vi "main.vi"() -> ()   [LabVIEW 2015]
uses:
  <vilib>/Utility/error.llb/DialogType.ctl
panel:
  out "d1_B2n":dbl
  out "d1_B1n":dbl
  out "d1_A2n":dbl
  out "d1_A1n":dbl
  out "con1":refnum<k5>
  in  "Tab Control":enum32{"ИЗМЕРЕНИЯ", "НАСТРОЙКИ"}(tab)
  out "d1_A1":string="-"
  out "d1_A2":string
  out "d1_B1":string="-"
  out "d1_B2":string
  in  "1_A1":bool=TRUE
  in  "1_A2":bool=TRUE
  in  "1_B1":bool=TRUE
  in  "1_B2":bool=TRUE
  out "con status 1":bool
  out "con2":refnum<k5>
  out "con status 2":bool
  in  "2_B1":bool=TRUE
  out "d2_B1":string="\r\n"
  in  "2_B2":bool=TRUE
  out "d2_B2":string="\r\n"
  in  "2_A2":bool=TRUE
  out "d2_A2":string
  in  "2_A1":bool=TRUE
  out "d2_A1":string
  out "d2_B2n":dbl
  out "d2_B1n":dbl
  out "d2_A2n":dbl
  out "d2_A1n":dbl
  out "refnum out":refnum<file>
  in  "P max lp":dbl=1000.0 min=0.0 max=10000000.0 step=1e-06 format="%3.2e"
  in  "P min lp":dbl min=0.0 max=10000000.0 step=1e-06 format="%3.2e"
  in  "Autoscale 2":bool=TRUE
  in  "P max hp":dbl=1000.0 min=0.0 max=10000000.0 step=1e-06 format="%3.2e"
  in  "P min hp":dbl min=0.0 max=10000000.0 step=1e-06 format="%3.2e"
  in  "Autoscale 1":bool=TRUE
  in  "port1":u16=4001
  in  "D1 IP":string="192.168.127.253"
  in  "D2 IP":string="192.168.127.253"
  in  "port2":u16=4001
  in  "d2_B2s":enum32{"Radio Selection 1", "Radio Selection 2"}(radio)
  in  "d2_B1s":enum32{"Radio Selection 1", "Radio Selection 2"}(radio)
  in  "d2_A2s":enum32{"Radio Selection 1", "Radio Selection 2"}(radio)
  in  "d2_A1s":enum32{"Radio Selection 1", "Radio Selection 2"}(radio)
  in  "d1_B2s":enum32{"Radio Selection 1", "Radio Selection 2"}(radio)
  in  "d1_B1s":enum32{"Radio Selection 1", "Radio Selection 2"}(radio)
  in  "d1_A2s":enum32{"Radio Selection 1", "Radio Selection 2"}(radio)
  in  "d1_A1s":enum32{"Radio Selection 1", "Radio Selection 2"}(radio)
  in  "stop":bool
  in  "xScale +":bool
  in  "xScale -":bool
  in  "Добавить время":dbl(ring)=300.0 items=["1 мин."=60.0, "5 мин."=300.0, "20 мин."=1200.0]
  out "мин.":string="1"
  out "часы":string="0"
  out "Graphs hP":dynamicdata(graph) caption="Высокий вакуум, мБар"
  out "сек.":string="0"
  out "Сутки":string
  out "Graphs lP":dynamicdata(graph) caption="Низкий вакуум, мБар"
  # "D1"
  # "A1"
  # "A2"
  # "B1"
  # "B2"
  # "D2"
  # "A1"
  # "A2"
  # "B1"
  # "B2"
  # "Высокий вакуум"
  # "Низкий вакуум"
  # "Отображение на графиках"
  # "Высокий"
  # "Низкий"
  # "D2 B2"
  # "D2 B1"
  # "D2 A2"
  # "D2 A1"
  # "D1 B2"
  # "D1 B1"
  # "D1 A2"
  # "D1 A1"
  # "Интервал графиков"
  # ":"
types:
  T1 = typedef "DialogType.ctl" = u16
  T2 = typedef "RWC_Actions.ctl" = enum16{"Read", "Write", "Read and Create"}
  T3 = typedef "LVDateTimeRec.ctl" = cluster{"fractional second":dbl, "second":i32, "minute":i32, "hour":i32, "day of month":i32, "month":i32, "year":i32, "day of week":i32, "day of year":i32, "DST":i32}
  T4 = enum8{"Enabled", "Disabled", "Disabled and Grayed Out"}
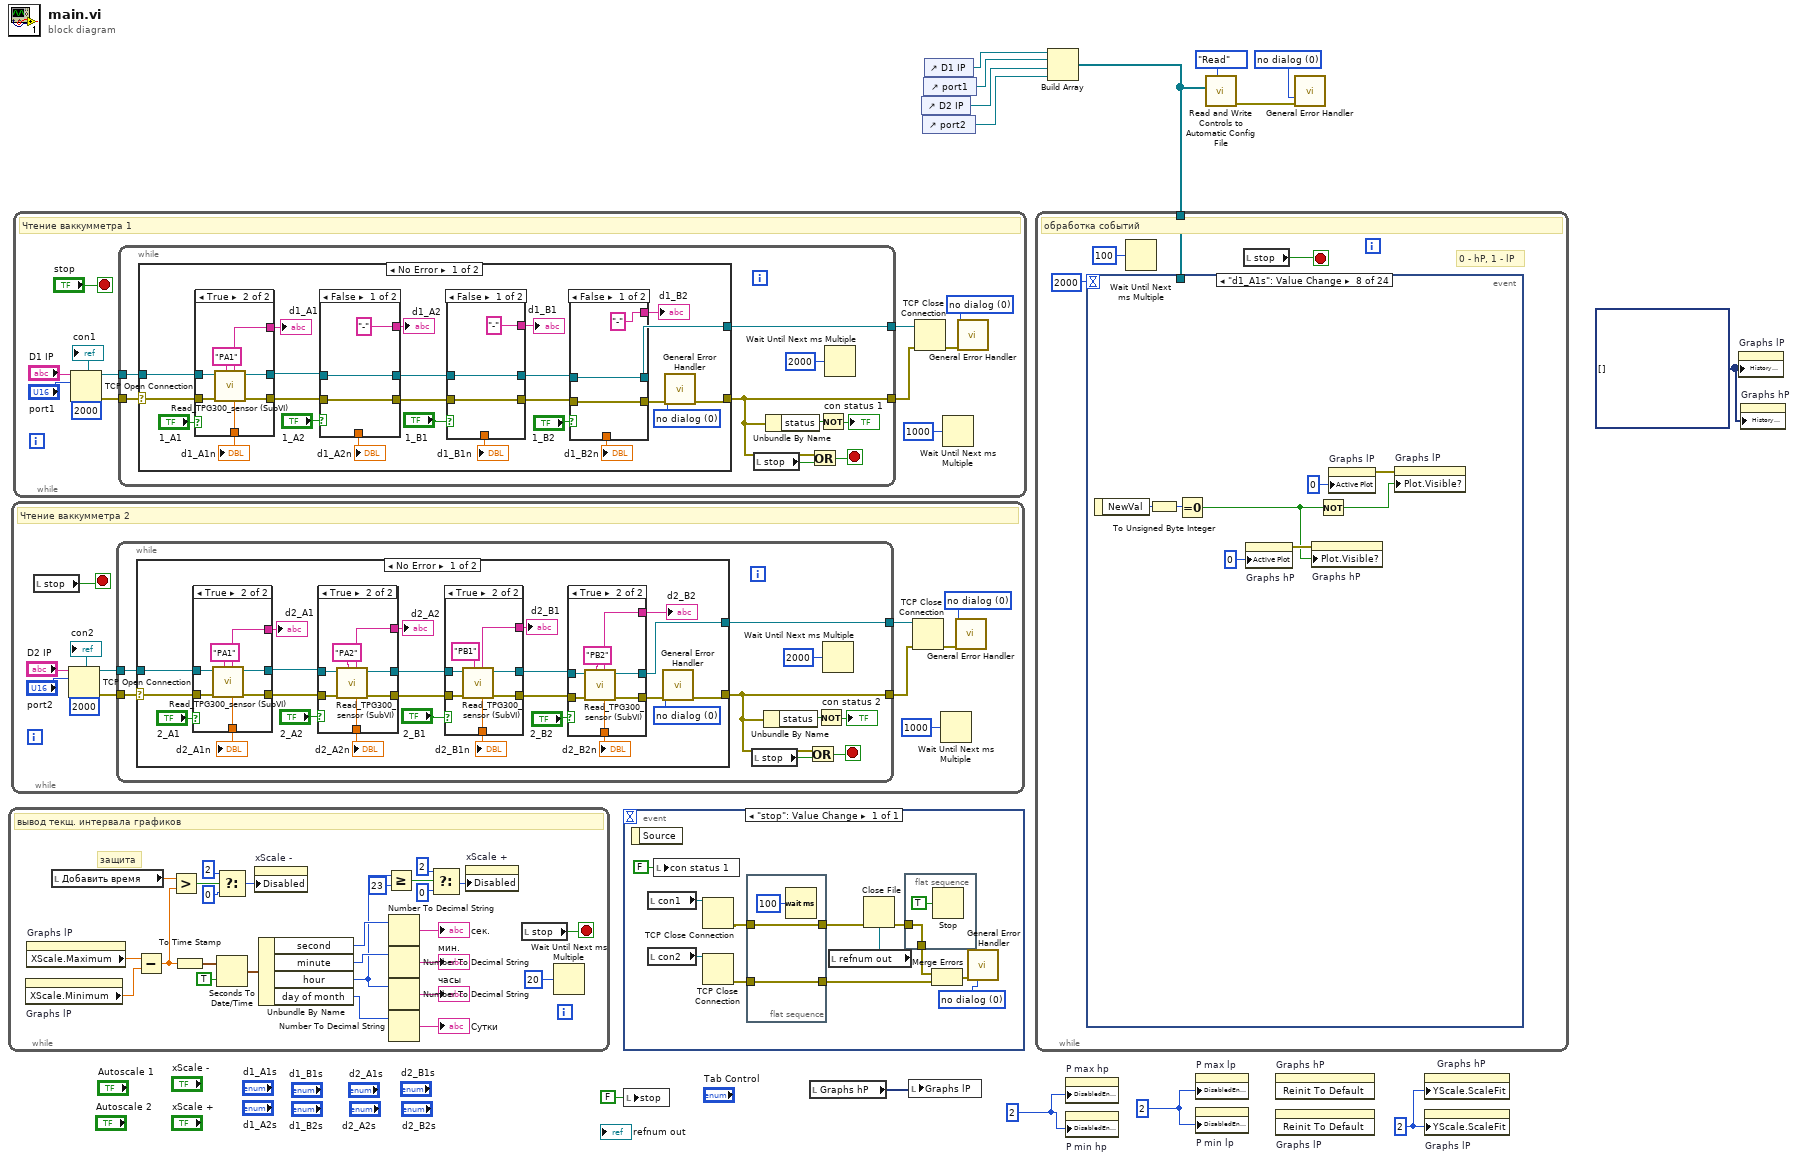
[diagram p0: block diagram]
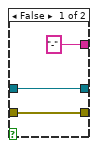
[diagram p2: hidden frame]
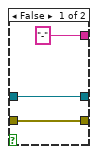
[diagram p3: hidden frame]
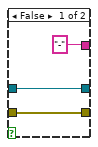
[diagram p4: hidden frame]
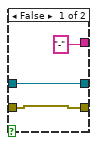
[diagram p5: hidden frame]
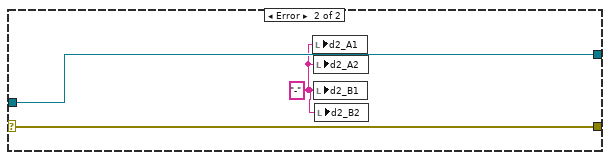
[diagram p6: hidden frame]
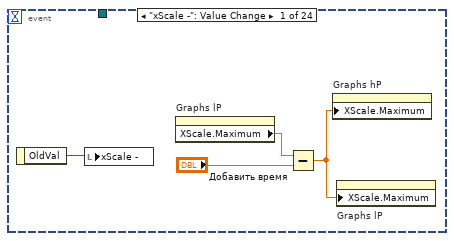
[diagram p7: hidden frame]
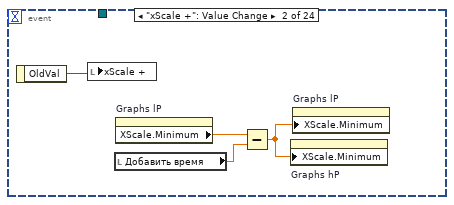
[diagram p8: hidden frame]
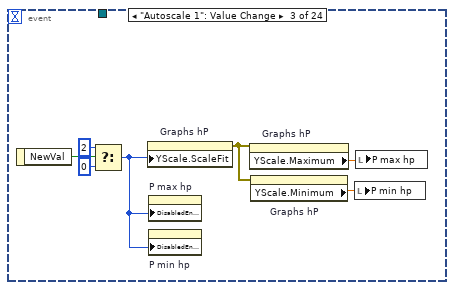
[diagram p9: hidden frame]
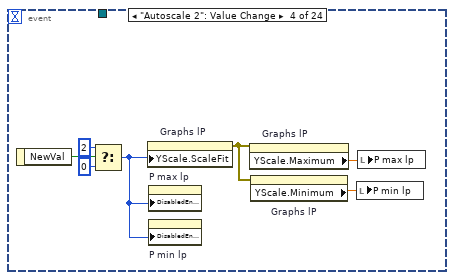
[diagram p10: hidden frame]
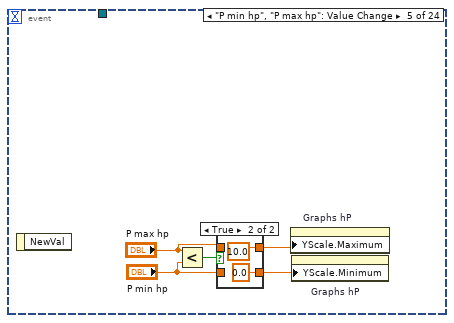
[diagram p11: hidden frame]
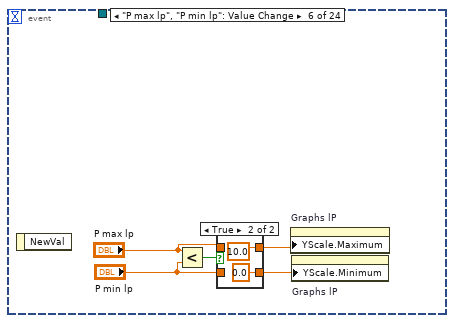
[diagram p13: hidden frame]
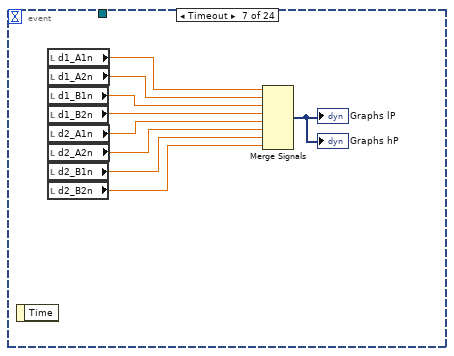
[diagram p15: hidden frame]
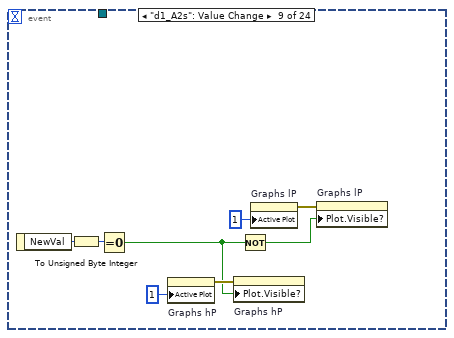
[diagram p16: hidden frame]
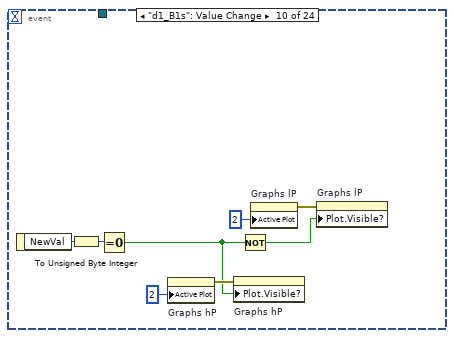
[diagram p17: hidden frame]
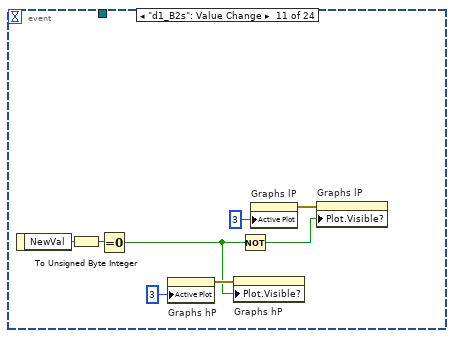
[diagram p18: hidden frame]
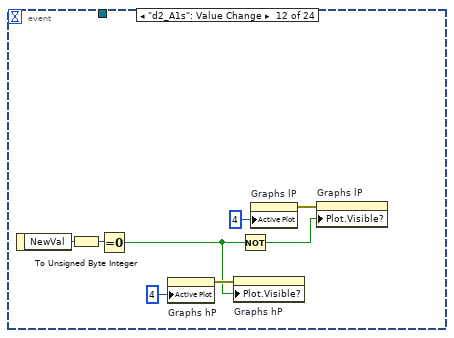
[diagram p19: hidden frame]
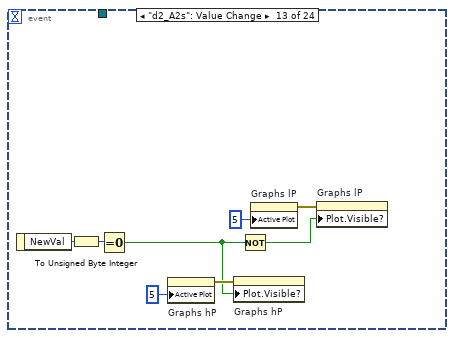
[diagram p20: hidden frame]
diagram:
  w6 = T1 0 items=["no dialog", "OK message", "continue or stop message", "OK message + warnings", "continue/stop + warnings"] ("type of dialog (OK msg:1)")
  w9 = u8 2 ("Y Scale.Scale Fit")
  w10 = u8 2 ("Y Scale.Scale Fit")
  w11 = u8 2 ("Y Scale.Scale Fit")
  w12 = dynamicdata[] [] ("History Data")
  n1 = while {
    stop <- w28 stop-if-true
    # "защита"
    # "вывод текщ. интервала графиков"
    n2 = property on="Graphs lP" class="WFChart (strict)"() -> ("XScale.Minimum"=w15:dbl)  [unwired: 2 in, 2 out]
    n3 = property on="Graphs lP" class="WFChart (strict)"() -> ("XScale.Maximum"=w16:dbl)  [unwired: 2 in, 2 out]
    n4 = local read "Добавить время"() -> (w40:dbl)
    n5 = Subtract(x=w16, y=w15) -> (x-y=w29:dbl)
    n6 = Greater?(x=w40, y=w29) -> (0:w26:bool)
    n7 = To Time Stamp(1:w29) -> (0:w38:timestamp)
    n8 = Select(t=u8 2 ("Disabled"), s=w26, f=u8 0 ("Disabled")) -> (s? t:f=w23:u8)
    n9 = Seconds To Date/Time(time stamp (now)=w38, to UTC (F)=TRUE) -> (date time rec=w37:T3)
    n10 = property on="xScale -" class="Bool (strict)"("Disabled"=w23) -> ()  [unwired: 2 in, 2 out]
    n11 = Unbundle By Name(w37) -> ("second"=w36:i32, "minute"=w35:i32, "hour"=w18:i32, "day of month"=w34:i32)
    n12 = Greater Or Equal?(x=w18, y=23) -> (x >= y?=w19:bool)
    n13 = Number To Decimal String(number=w36) -> (decimal integer string=→"сек.":string)  [unwired: 1 out]
    n14 = Number To Decimal String(number=w35) -> (decimal integer string=→"мин.":string)  [unwired: 1 out]
    n15 = Number To Decimal String(number=w18) -> (decimal integer string=→"часы":string)  [unwired: 1 out]
    n16 = Number To Decimal String(number=w34) -> (decimal integer string=→"Сутки":string)  [unwired: 1 out]
    n17 = Select(t=u8 2 ("Disabled"), s=w19, f=u8 0 ("Disabled")) -> (s? t:f=w17:u8)
    n18 = property on="xScale +" class="Bool (strict)"("Disabled"=w17) -> ()  [unwired: 2 in, 2 out]
    n19 = local read "stop"() -> (w28:bool)
    n20 = Wait Until Next ms Multiple(millisecond multiple=u32 20) -> ()  [unwired: 1 out]
  }
  n21 = while {
    stop <- w41 stop-if-true
    w46 = T1 0 items=["no dialog", "OK message", "continue or stop message", "OK message + warnings", "continue/stop + warnings"] ("type of dialog (OK msg:1)")
    # "Чтение ваккумметра 2"
    n22 = local read "stop"() -> (w41:bool)
    n23 = TCP Open Connection(address="D2 IP", remote port or service name="port2", timeout ms (60000)=2000) -> (connection ID=w50:refnum<k5>, error out=w49:errorcluster)  [unwired: 1 in, 1 out]
    "con2" <- w50
    n24 = while {
      tunnel: w50 -> [w59]
      tunnel: w49 -> [w58]
      tunnel: [w60] -> w47
      tunnel: [w53] -> w44
      stop <- w55 stop-if-true
      n25 = case shown="No Error" w58 {
        selector: w58 -> [w84 w126]
        tunnel: w59 -> [w83 w127]
        tunnel: [w77 w127] -> w60
        tunnel: [w80 w126] -> w53
        frame No Error {
          w82 = T1 0 items=["no dialog", "OK message", "continue or stop message", "OK message + warnings", "continue/stop + warnings"] ("type of dialog (OK msg:1)")
          n26 = case shown="True" "2_A1" {
            tunnel: w84 -> [w116 w120]
            tunnel: w83 -> [w117 w124]
            tunnel: [w116 w122] -> w74
            tunnel: [w117 w121] -> w75
            tunnel: [_ w118] -> w68
            tunnel: ["-" ("A1") w119] -> w64
            frame False {
            }
            frame True {
              n27 = call "Read_TPG300_sensor (SubVI).vi"("Sensor CMD"="PA1" ("data in"), "error in (no error)"=w120, "TCP Network Connection in"=w124) -> ("error out"=w122:errorcluster, "connection ID out"=w121:refnum<k5>, "out number"=w118:dbl, "data out"=w119:string)  [unwired: 5 in]
            }
          }
          "d2_A1n" <- w68
          "d2_A1" <- w64
          n28 = case shown="True" "2_A2" {
            tunnel: [w107 w114] -> w72
            tunnel: [w106 w113] -> w71
            tunnel: w75 -> [w107 w111]
            tunnel: w74 -> [w106 w110]
            tunnel: [_ w108] -> w67
            tunnel: ["-" ("A2") w109] -> w63
            frame False {
            }
            frame True {
              n29 = call "Read_TPG300_sensor (SubVI).vi"("Sensor CMD"="PA2" ("data in"), "error in (no error)"=w110, "TCP Network Connection in"=w111) -> ("error out"=w113:errorcluster, "connection ID out"=w114:refnum<k5>, "out number"=w108:dbl, "data out"=w109:string)  [unwired: 5 in]
            }
          }
          "d2_A2n" <- w67
          "d2_A2" <- w63
          n30 = case shown="True" "2_B1" {
            tunnel: w71 -> [w86 w93]
            tunnel: w72 -> [w87 w92]
            tunnel: [w86 w91] -> w69
            tunnel: [w87 w90] -> w70
            tunnel: [_ w88] -> w66
            tunnel: ["-" ("B1") w89] -> w62
            frame False {
            }
            frame True {
              n31 = call "Read_TPG300_sensor (SubVI).vi"("Sensor CMD"="PB1" ("data in"), "error in (no error)"=w93, "TCP Network Connection in"=w92) -> ("error out"=w91:errorcluster, "connection ID out"=w90:refnum<k5>, "out number"=w88:dbl, "data out"=w89:string)  [unwired: 5 in]
            }
          }
          "d2_B1n" <- w66
          "d2_B1" <- w62
          n32 = case shown="True" "2_B2" {
            tunnel: w69 -> [w97 w103]
            tunnel: w70 -> [w96 w102]
            tunnel: [_ w98] -> w65
            tunnel: [w97 w101] -> w76
            tunnel: [w96 w100] -> w77
            tunnel: ["-" ("B2") w99] -> w61
            frame False {
            }
            frame True {
              n33 = call "Read_TPG300_sensor (SubVI).vi"("Sensor CMD"="PB2" ("data in"), "error in (no error)"=w103, "TCP Network Connection in"=w102) -> ("error out"=w101:errorcluster, "connection ID out"=w100:refnum<k5>, "out number"=w98:dbl, "data out"=w99:string)  [unwired: 5 in]
            }
          }
          "d2_B2n" <- w65
          "d2_B2" <- w61
          n34 = call <vilib>:"General Error Handler.vi"("type of dialog (OK msg:1)"=w82, "error in (no error)"=w76) -> ("error out"=w80:errorcluster)  [unwired: 9 in, 4 out]
        }
        frame Error {
          w125 = "-" ("d2_B1")
          n35 = local write "d2_A1"(w125) -> ()
          n36 = local write "d2_A2"(w125) -> ()
          n37 = local write "d2_B1"(w125) -> ()
          n38 = local write "d2_B2"(w125) -> ()
        }
      }
      n39 = local read "stop"() -> (w52:bool)
      n40 = Unbundle By Name(w53) -> ("status"=w57:bool)
      n41 = Or(x=w53, y=w52) -> (x .or. y?=w55:bool)
      n42 = Not(x=w57) -> (.not. x?=→"con status 2":bool)
      n43 = Wait Until Next ms Multiple(millisecond multiple=u32 2000) -> ()  [unwired: 1 out]
    }
    n44 = TCP Close Connection(connection ID=w47, error in (no error)=w44) -> (error out=w45:errorcluster)  [unwired: 1 in, 1 out]
    n45 = Wait Until Next ms Multiple(millisecond multiple=u32 1000) -> ()  [unwired: 1 out]
    n46 = call <vilib>:"General Error Handler.vi"("type of dialog (OK msg:1)"=w46, "error in (no error)"=w45) -> ()  [unwired: 9 in, 5 out]
  }
  n47 = while {
    stop <- "stop" stop-if-true
    w133 = T1 0 items=["no dialog", "OK message", "continue or stop message", "OK message + warnings", "continue/stop + warnings"] ("type of dialog (OK msg:1)")
    # "Чтение ваккумметра 1"
    n48 = TCP Open Connection(address="D1 IP", remote port or service name="port1", timeout ms (60000)=2000) -> (connection ID=w137:refnum<k5>, error out=w136:errorcluster)  [unwired: 1 in, 1 out]
    "con1" <- w137
    n49 = while {
      tunnel: w137 -> [w146]
      tunnel: w136 -> [w145]
      tunnel: [w147] -> w134
      tunnel: [w139] -> w131
      stop <- w141 stop-if-true
      n50 = case shown="No Error" w145 {
        selector: w145 -> [w171 w214]
        tunnel: w146 -> [w170 w215]
        tunnel: [w164 w215] -> w147
        tunnel: [w167 w214] -> w139
        frame No Error {
          w169 = T1 0 items=["no dialog", "OK message", "continue or stop message", "OK message + warnings", "continue/stop + warnings"] ("type of dialog (OK msg:1)")
          n51 = case shown="True" "1_A1" {
            tunnel: w171 -> [w203 w207]
            tunnel: w170 -> [w204 w211]
            tunnel: [w203 w209] -> w161
            tunnel: [w204 w208] -> w162
            tunnel: [_ w205] -> w155
            tunnel: ["-" ("A1") w206] -> w151
            frame False {
            }
            frame True {
              n52 = call "Read_TPG300_sensor (SubVI).vi"("Sensor CMD"="PA1" ("data in"), "error in (no error)"=w207, "TCP Network Connection in"=w211) -> ("error out"=w209:errorcluster, "connection ID out"=w208:refnum<k5>, "out number"=w205:dbl, "data out"=w206:string)  [unwired: 5 in]
            }
          }
          "d1_A1n" <- w155
          "d1_A1" <- w151
          n53 = case shown="False" "1_A2" {
            tunnel: [w194 w201] -> w159
            tunnel: [w193 w200] -> w158
            tunnel: w162 -> [w194 w198]
            tunnel: w161 -> [w193 w197]
            tunnel: [_ w195] -> w154
            tunnel: ["-" ("A2") w196] -> w150
            frame False {
            }
            frame True {
              n54 = call "Read_TPG300_sensor (SubVI).vi"("Sensor CMD"="PA2" ("data in"), "error in (no error)"=w197, "TCP Network Connection in"=w198) -> ("error out"=w200:errorcluster, "connection ID out"=w201:refnum<k5>, "out number"=w195:dbl, "data out"=w196:string)  [unwired: 5 in]
            }
          }
          "d1_A2n" <- w154
          "d1_A2" <- w150
          n55 = case shown="False" "1_B1" {
            tunnel: w158 -> [w173 w180]
            tunnel: w159 -> [w174 w179]
            tunnel: [w173 w178] -> w156
            tunnel: [w174 w177] -> w157
            tunnel: [_ w176] -> w153
            tunnel: ["-" ("B1") w175] -> w149
            frame False {
            }
            frame True {
              n56 = call "Read_TPG300_sensor (SubVI).vi"("Sensor CMD"="PB1" ("data in"), "error in (no error)"=w180, "TCP Network Connection in"=w179) -> ("error out"=w178:errorcluster, "connection ID out"=w177:refnum<k5>, "out number"=w176:dbl, "data out"=w175:string)  [unwired: 5 in]
            }
          }
          "d1_B1n" <- w153
          "d1_B1" <- w149
          n57 = case shown="False" "1_B2" {
            tunnel: w156 -> [w184 w190]
            tunnel: w157 -> [w183 w189]
            tunnel: [_ w185] -> w152
            tunnel: [w184 w188] -> w163
            tunnel: [w183 w187] -> w164
            tunnel: ["-" ("B2") w186] -> w148
            frame False {
            }
            frame True {
              n58 = call "Read_TPG300_sensor (SubVI).vi"("Sensor CMD"="PB2" ("data in"), "error in (no error)"=w190, "TCP Network Connection in"=w189) -> ("error out"=w188:errorcluster, "connection ID out"=w187:refnum<k5>, "out number"=w185:dbl, "data out"=w186:string)  [unwired: 5 in]
            }
          }
          "d1_B2n" <- w152
          "d1_B2" <- w148
          n59 = call <vilib>:"General Error Handler.vi"("type of dialog (OK msg:1)"=w169, "error in (no error)"=w163) -> ("error out"=w167:errorcluster)  [unwired: 9 in, 4 out]
        }
        frame Error {
          w212 = "-" ("d2_B1")
          w213 = "-" ("d2_B1")
          n60 = local write "d1_A1"(w213) -> ()
          n61 = local write "d1_A2"(w213) -> ()
          n62 = local write "d1_B1"(w212) -> ()
          n63 = local write "d1_B2"(w212) -> ()
        }
      }
      n64 = local read "stop"() -> (w142:bool)
      n65 = Unbundle By Name(w139) -> ("status"=w144:bool)
      n66 = Or(x=w139, y=w142) -> (x .or. y?=w141:bool)
      n67 = Not(x=w144) -> (.not. x?=→"con status 1":bool)
      n68 = Wait Until Next ms Multiple(millisecond multiple=u32 2000) -> ()  [unwired: 1 out]
    }
    n69 = TCP Close Connection(connection ID=w134, error in (no error)=w131) -> (error out=w132:errorcluster)  [unwired: 1 in, 1 out]
    n70 = Wait Until Next ms Multiple(millisecond multiple=u32 1000) -> ()  [unwired: 1 out]
    n71 = call <vilib>:"General Error Handler.vi"("type of dialog (OK msg:1)"=w133, "error in (no error)"=w132) -> ()  [unwired: 9 in, 5 out]
  }
  n72 = event shown="[0] \"stop\": Value Change" {
    selector: _ -> [_]
    dyn-events: _ -> [_]
    timeout: _ -> [_]
    event "stop": Value Change {
      w227 = T1 0 items=["no dialog", "OK message", "continue or stop message", "OK message + warnings", "continue/stop + warnings"] ("type of dialog (OK msg:1)")
      n73 = event-data() -> ()  [unwired: 1 in, 1 out]
      n74 = local read "con1"() -> (w222:refnum<k5>)
      n75 = local read "con2"() -> (w220:refnum<k5>)
      n76 = local write "con status 1"(FALSE ("con status")) -> ()
      n77 = TCP Close Connection(connection ID=w222) -> (error out=w223:errorcluster)  [unwired: 2 in, 1 out]
      n78 = TCP Close Connection(connection ID=w220) -> (error out=w219:errorcluster)  [unwired: 2 in, 1 out]
      n79 = flat-sequence {
        tunnel: [w231] -> w226
        tunnel: w223 -> [w231]
        tunnel: [w230] -> w218
        tunnel: w219 -> [w230]
        frame #0 {
          n80 = Wait (ms)(milliseconds to wait=u32 100) -> ()  [unwired: 1 out]
        }
      }
      n81 = local read "refnum out"() -> (w221:refnum<file>)
      n82 = Close File(refnum=w221, error in=w226) -> (error out=w225:errorcluster)  [unwired: 1 out]
      n83 = flat-sequence {
        tunnel: w225 -> [w228]
        tunnel: [w228] -> w217
        frame #0 {
          n84 = Stop(stop? (T)=TRUE) -> ()
        }
      }
      n85 = Merge Errors(w217, w218) -> (w216:errorcluster)
      n86 = call <vilib>:"General Error Handler.vi"("error in (no error)"=w216, "[exception action] (none:0)"=w227) -> ()  [unwired: 2 in, 12 out]
    }
  }
  n87 = local write "stop"(FALSE ("stop")) -> ()
  n88 = local read "Graphs hP"() -> (w13:dynamicdata)
  n89 = local write "Graphs lP"(w13) -> ()
  n90 = control-ref of="D2 IP"() -> (w3:refnum<vi>)
  n91 = control-ref of="port2"() -> (w2:refnum<vi>)
  n92 = control-ref of="port1"() -> (w4:refnum<vi>)
  n93 = control-ref of="D1 IP"() -> (w5:refnum<vi>)
  n94 = Build Array(w5, w4, w3, w2) -> (w1:refnum<vi>[])
  n95 = while {
    tunnel: w1 -> [w233]
    stop <- w236 stop-if-true
    # "0 - hP, 1 - lP"
    # "обработка событий"
    n96 = event shown="[7] \"d1_A1s\": Value Change" {
      selector: _ -> [_ _ _ _ _ _ _ _ _ _ _ _ _ _ _ _ _ _ _ _ _ _ _ _]
      dyn-events: _ -> [_ _ _ _ _ _ _ _ _ _ _ _ _ _ _ _ _ _ _ _ _ _ _ _]
      timeout: 2000 -> [_ _ _ _ _ _ _ _ _ _ _ _ _ _ _ _ _ _ _ _ _ _ _ _]
      tunnel: w233 -> [_ _ _ _ _ _ _ _ _ _ _ _ _ _ _ _ _ _ _ _ _ _ _ w432]
      event "xScale -": Value Change {
        n97 = event-data() -> ("OldVal"=w240:bool)  [unwired: 1 in]
        n98 = local write "xScale -"(w240) -> ()
        n99 = property on="Graphs lP" class="WFChart (strict)"() -> ("XScale.Maximum"=w238:dbl)  [unwired: 2 in, 2 out]
        n100 = Subtract(x=w238, y="Добавить время") -> (x-y=w237:dbl)
        n101 = property on="Graphs hP" class="WFChart (strict)"("XScale.Maximum"=w237) -> ()  [unwired: 2 in, 2 out]
        n102 = property on="Graphs lP" class="WFChart (strict)"("XScale.Maximum"=w237) -> ()  [unwired: 2 in, 2 out]
      }
      event "xScale +": Value Change {
        n103 = event-data() -> ("OldVal"=w244:bool)  [unwired: 1 in]
        n104 = local write "xScale +"(w244) -> ()
        n105 = local read "Добавить время"() -> (w243:dbl)
        n106 = property on="Graphs lP" class="WFChart (strict)"() -> ("XScale.Minimum"=w242:dbl)  [unwired: 2 in, 2 out]
        n107 = Subtract(x=w242, y=w243) -> (x-y=w241:dbl)
        n108 = property on="Graphs hP" class="WFChart (strict)"("XScale.Minimum"=w241) -> ()  [unwired: 2 in, 2 out]
        n109 = property on="Graphs lP" class="WFChart (strict)"("XScale.Minimum"=w241) -> ()  [unwired: 2 in, 2 out]
      }
      event "Autoscale 1": Value Change {
        n110 = event-data() -> ("NewVal"=w251:bool)  [unwired: 1 in]
        n111 = Select(t=u8 2 ("Y Scale.Scale Fit"), s=w251, f=u8 0 ("Y Scale.Scale Fit")) -> (s? t:f=w248:u8)
        n112 = property on="Graphs hP" class="WFChart (strict)"("YScale.ScaleFit"=w248) -> (error out=w247:errorcluster)  [unwired: 2 in, 1 out]
        n113 = property on="P max hp" class="DigNum (strict)"("DisabledEnum"=w248) -> ()  [unwired: 2 in, 2 out]
        n114 = property on="P min hp" class="DigNum (strict)"("DisabledEnum"=w248) -> ()  [unwired: 2 in, 2 out]
        n115 = property on="Graphs hP" class="WFChart (strict)"(error in=w247) -> ("YScale.Maximum"=w245:dbl)  [unwired: 1 in, 2 out]
        n116 = property on="Graphs hP" class="WFChart (strict)"(error in=w247) -> ("YScale.Minimum"=w246:dbl)  [unwired: 1 in, 2 out]
        n117 = local write "P min hp"(w246) -> ()
        n118 = local write "P max hp"(w245) -> ()
      }
      event "Autoscale 2": Value Change {
        n119 = event-data() -> ("NewVal"=w258:bool)  [unwired: 1 in]
        n120 = Select(t=u8 2 ("Y Scale.Scale Fit"), s=w258, f=u8 0 ("Y Scale.Scale Fit")) -> (s? t:f=w255:u8)
        n121 = property on="Graphs lP" class="WFChart (strict)"("YScale.ScaleFit"=w255) -> (error out=w254:errorcluster)  [unwired: 2 in, 1 out]
        n122 = property on="P max lp" class="DigNum (strict)"("DisabledEnum"=w255) -> ()  [unwired: 2 in, 2 out]
        n123 = property on="P min lp" class="DigNum (strict)"("DisabledEnum"=w255) -> ()  [unwired: 2 in, 2 out]
        n124 = property on="Graphs lP" class="WFChart (strict)"(error in=w254) -> ("YScale.Maximum"=w252:dbl)  [unwired: 1 in, 2 out]
        n125 = property on="Graphs lP" class="WFChart (strict)"(error in=w254) -> ("YScale.Minimum"=w253:dbl)  [unwired: 1 in, 2 out]
        n126 = local write "P min lp"(w253) -> ()
        n127 = local write "P max lp"(w252) -> ()
      }
      event "P min hp", "P max hp": Value Change {
        n128 = event-data() -> ()  [unwired: 1 in, 1 out]
        n129 = Less?(x="P max hp", y="P min hp") -> (x < y?=w263:bool)
        n130 = case shown="True" w263 {
          tunnel: [w264 10.0 ("x+1")] -> w260
          tunnel: [w265 0.0 ("x+1")] -> w259
          tunnel: "P max hp" -> [w264 _]
          tunnel: "P min hp" -> [w265 _]
          frame False {
          }
          frame True {
          }
        }
        n131 = property on="Graphs hP" class="WFChart (strict)"("YScale.Maximum"=w260) -> ()  [unwired: 2 in, 2 out]
        n132 = property on="Graphs hP" class="WFChart (strict)"("YScale.Minimum"=w259) -> ()  [unwired: 2 in, 2 out]
      }
      event "P max lp", "P min lp": Value Change {
        n133 = event-data() -> ()  [unwired: 1 in, 1 out]
        n134 = Less?(x="P max lp", y="P min lp") -> (x < y?=w272:bool)
        n135 = case shown="True" w272 {
          tunnel: [w273 10.0 ("x+1")] -> w271
          tunnel: [w274 0.0 ("x+1")] -> w270
          tunnel: "P max lp" -> [w273 _]
          tunnel: "P min lp" -> [w274 _]
          frame False {
          }
          frame True {
          }
        }
        n136 = property on="Graphs lP" class="WFChart (strict)"("YScale.Maximum"=w271) -> ()  [unwired: 2 in, 2 out]
        n137 = property on="Graphs lP" class="WFChart (strict)"("YScale.Minimum"=w270) -> ()  [unwired: 2 in, 2 out]
      }
      event Timeout {
        # "0 - hP, 1 - lP"
        n138 = event-data() -> ()  [unwired: 1 in, 1 out]
        n139 = local read "d1_A1n"() -> (w278:dbl)
        n140 = local read "d1_A2n"() -> (w279:dbl)
        n141 = local read "d1_B1n"() -> (w280:dbl)
        n142 = local read "d1_B2n"() -> (w281:dbl)
        n143 = local read "d2_A1n"() -> (w282:dbl)
        n144 = local read "d2_A2n"() -> (w283:dbl)
        n145 = local read "d2_B1n"() -> (w284:dbl)
        n146 = local read "d2_B2n"() -> (w285:dbl)
        n147 = Merge Signals(w278, w279, w280, w281, w282, w283, w284, w285) -> (→"Graphs lP" →"Graphs hP":dynamicdata)
      }
      event "d1_A1s": Value Change {
        n148 = event-data() -> ("NewVal"=w289:enum32{"Radio Selection 1", "Radio Selection 2"})  [unwired: 1 in]
        n149 = To Unsigned Byte Integer(number=w289) -> (unsigned 8bit integer=w288:u8)
        n150 = Equal To 0?(x=w288) -> (x = 0?=w287:bool)
        n151 = property on="Graphs hP" class="WFChart (strict)"("Active Plot"=u32 0) -> (error out=w293:errorcluster)  [unwired: 2 in, 1 out]
        n152 = property on="Graphs hP" class="WFChart (strict)"(error in=w293, "Plot.Visible?"=w287) -> ()  [unwired: 1 in, 2 out]
        n153 = Not(x=w287) -> (.not. x?=w286:bool)
        n154 = property on="Graphs lP" class="WFChart (strict)"("Active Plot"=u32 0) -> (error out=w290:errorcluster)  [unwired: 2 in, 1 out]
        n155 = property on="Graphs lP" class="WFChart (strict)"(error in=w290, "Plot.Visible?"=w286) -> ()  [unwired: 1 in, 2 out]
      }
      event "d1_A2s": Value Change {
        n156 = event-data() -> ("NewVal"=w297:enum32{"Radio Selection 1", "Radio Selection 2"})  [unwired: 1 in]
        n157 = To Unsigned Byte Integer(number=w297) -> (unsigned 8bit integer=w296:u8)
        n158 = Equal To 0?(x=w296) -> (x = 0?=w295:bool)
        n159 = property on="Graphs hP" class="WFChart (strict)"("Active Plot"=u32 1) -> (error out=w301:errorcluster)  [unwired: 2 in, 1 out]
        n160 = property on="Graphs hP" class="WFChart (strict)"(error in=w301, "Plot.Visible?"=w295) -> ()  [unwired: 1 in, 2 out]
        n161 = Not(x=w295) -> (.not. x?=w294:bool)
        n162 = property on="Graphs lP" class="WFChart (strict)"("Active Plot"=u32 1) -> (error out=w298:errorcluster)  [unwired: 2 in, 1 out]
        n163 = property on="Graphs lP" class="WFChart (strict)"(error in=w298, "Plot.Visible?"=w294) -> ()  [unwired: 1 in, 2 out]
      }
      event "d1_B1s": Value Change {
        n164 = event-data() -> ("NewVal"=w305:enum32{"Radio Selection 1", "Radio Selection 2"})  [unwired: 1 in]
        n165 = To Unsigned Byte Integer(number=w305) -> (unsigned 8bit integer=w304:u8)
        n166 = Equal To 0?(x=w304) -> (x = 0?=w303:bool)
        n167 = property on="Graphs hP" class="WFChart (strict)"("Active Plot"=u32 2) -> (error out=w309:errorcluster)  [unwired: 2 in, 1 out]
        n168 = property on="Graphs hP" class="WFChart (strict)"(error in=w309, "Plot.Visible?"=w303) -> ()  [unwired: 1 in, 2 out]
        n169 = Not(x=w303) -> (.not. x?=w302:bool)
        n170 = property on="Graphs lP" class="WFChart (strict)"("Active Plot"=u32 2) -> (error out=w306:errorcluster)  [unwired: 2 in, 1 out]
        n171 = property on="Graphs lP" class="WFChart (strict)"(error in=w306, "Plot.Visible?"=w302) -> ()  [unwired: 1 in, 2 out]
      }
      event "d1_B2s": Value Change {
        n172 = event-data() -> ("NewVal"=w313:enum32{"Radio Selection 1", "Radio Selection 2"})  [unwired: 1 in]
        n173 = To Unsigned Byte Integer(number=w313) -> (unsigned 8bit integer=w312:u8)
        n174 = Equal To 0?(x=w312) -> (x = 0?=w311:bool)
        n175 = property on="Graphs hP" class="WFChart (strict)"("Active Plot"=u32 3) -> (error out=w317:errorcluster)  [unwired: 2 in, 1 out]
        n176 = property on="Graphs hP" class="WFChart (strict)"(error in=w317, "Plot.Visible?"=w311) -> ()  [unwired: 1 in, 2 out]
        n177 = Not(x=w311) -> (.not. x?=w310:bool)
        n178 = property on="Graphs lP" class="WFChart (strict)"("Active Plot"=u32 3) -> (error out=w314:errorcluster)  [unwired: 2 in, 1 out]
        n179 = property on="Graphs lP" class="WFChart (strict)"(error in=w314, "Plot.Visible?"=w310) -> ()  [unwired: 1 in, 2 out]
      }
      event "d2_A1s": Value Change {
        n180 = event-data() -> ("NewVal"=w321:enum32{"Radio Selection 1", "Radio Selection 2"})  [unwired: 1 in]
        n181 = To Unsigned Byte Integer(number=w321) -> (unsigned 8bit integer=w320:u8)
        n182 = Equal To 0?(x=w320) -> (x = 0?=w319:bool)
        n183 = property on="Graphs hP" class="WFChart (strict)"("Active Plot"=u32 4) -> (error out=w325:errorcluster)  [unwired: 2 in, 1 out]
        n184 = property on="Graphs hP" class="WFChart (strict)"(error in=w325, "Plot.Visible?"=w319) -> ()  [unwired: 1 in, 2 out]
        n185 = Not(x=w319) -> (.not. x?=w318:bool)
        n186 = property on="Graphs lP" class="WFChart (strict)"("Active Plot"=u32 4) -> (error out=w322:errorcluster)  [unwired: 2 in, 1 out]
        n187 = property on="Graphs lP" class="WFChart (strict)"(error in=w322, "Plot.Visible?"=w318) -> ()  [unwired: 1 in, 2 out]
      }
      event "d2_A2s": Value Change {
        n188 = event-data() -> ("NewVal"=w329:enum32{"Radio Selection 1", "Radio Selection 2"})  [unwired: 1 in]
        n189 = To Unsigned Byte Integer(number=w329) -> (unsigned 8bit integer=w328:u8)
        n190 = Equal To 0?(x=w328) -> (x = 0?=w327:bool)
        n191 = property on="Graphs hP" class="WFChart (strict)"("Active Plot"=u32 5) -> (error out=w333:errorcluster)  [unwired: 2 in, 1 out]
        n192 = property on="Graphs hP" class="WFChart (strict)"(error in=w333, "Plot.Visible?"=w327) -> ()  [unwired: 1 in, 2 out]
        n193 = Not(x=w327) -> (.not. x?=w326:bool)
        n194 = property on="Graphs lP" class="WFChart (strict)"("Active Plot"=u32 5) -> (error out=w330:errorcluster)  [unwired: 2 in, 1 out]
        n195 = property on="Graphs lP" class="WFChart (strict)"(error in=w330, "Plot.Visible?"=w326) -> ()  [unwired: 1 in, 2 out]
      }
      event "d2_B1s": Value Change {
        n196 = event-data() -> ("NewVal"=w337:enum32{"Radio Selection 1", "Radio Selection 2"})  [unwired: 1 in]
        n197 = To Unsigned Byte Integer(number=w337) -> (unsigned 8bit integer=w336:u8)
        n198 = Equal To 0?(x=w336) -> (x = 0?=w335:bool)
        n199 = property on="Graphs hP" class="WFChart (strict)"("Active Plot"=u32 6) -> (error out=w341:errorcluster)  [unwired: 2 in, 1 out]
        n200 = property on="Graphs hP" class="WFChart (strict)"(error in=w341, "Plot.Visible?"=w335) -> ()  [unwired: 1 in, 2 out]
        n201 = Not(x=w335) -> (.not. x?=w334:bool)
        n202 = property on="Graphs lP" class="WFChart (strict)"("Active Plot"=u32 6) -> (error out=w338:errorcluster)  [unwired: 2 in, 1 out]
        n203 = property on="Graphs lP" class="WFChart (strict)"(error in=w338, "Plot.Visible?"=w334) -> ()  [unwired: 1 in, 2 out]
      }
      event "d2_B2s": Value Change {
        n204 = event-data() -> ("NewVal"=w345:enum32{"Radio Selection 1", "Radio Selection 2"})  [unwired: 1 in]
        n205 = To Unsigned Byte Integer(number=w345) -> (unsigned 8bit integer=w344:u8)
        n206 = Equal To 0?(x=w344) -> (x = 0?=w343:bool)
        n207 = property on="Graphs hP" class="WFChart (strict)"("Active Plot"=u32 7) -> (error out=w349:errorcluster)  [unwired: 2 in, 1 out]
        n208 = property on="Graphs hP" class="WFChart (strict)"(error in=w349, "Plot.Visible?"=w343) -> ()  [unwired: 1 in, 2 out]
        n209 = Not(x=w343) -> (.not. x?=w342:bool)
        n210 = property on="Graphs lP" class="WFChart (strict)"("Active Plot"=u32 7) -> (error out=w346:errorcluster)  [unwired: 2 in, 1 out]
        n211 = property on="Graphs lP" class="WFChart (strict)"(error in=w346, "Plot.Visible?"=w342) -> ()  [unwired: 1 in, 2 out]
      }
      event "1_A1": Value Change {
        n212 = event-data() -> ("NewVal"=w351:bool)  [unwired: 1 in]
        n213 = Select(t=T4."Enabled" ("Disabled"), s=w351, f=T4."Disabled and Grayed Out" ("Disabled")) -> (s? t:f=w350:T4)
        n214 = property on="d1_A1" class="Str"("DisabledEnum"=w350) -> ()  [unwired: 2 in, 2 out]
        n215 = property on="d1_A1s" class="RadioBtnsControl (strict)"("DisabledEnum"=w350) -> ()  [unwired: 2 in, 2 out]
        n216 = case shown="True" w351 {
          frame False {
            w354 = FALSE ("Plot.Visible")
            n217 = property on="Graphs hP" class="WFChart (strict)"("Active Plot"=u32 0) -> (error out=w358:errorcluster)  [unwired: 2 in, 1 out]
            n218 = property on="Graphs lP" class="WFChart (strict)"("Active Plot"=u32 0) -> (error out=w355:errorcluster)  [unwired: 2 in, 1 out]
            n219 = property on="Graphs hP" class="WFChart (strict)"(error in=w358, "Plot.Visible?"=w354) -> ()  [unwired: 1 in, 2 out]
            n220 = property on="Graphs lP" class="WFChart (strict)"(error in=w355, "Plot.Visible?"=w354) -> ()  [unwired: 1 in, 2 out]
          }
          frame True {
            n221 = local read "d1_A1s"() -> (w359:enum32{"Radio Selection 1", "Radio Selection 2"})
            n222 = property on="d1_A1s" class="RadioBtnsControl (strict)"("Val(Sgnl)"=w359) -> ()  [unwired: 2 in, 2 out]
          }
        }
      }
      event "1_A2": Value Change {
        n223 = event-data() -> ("NewVal"=w361:bool)  [unwired: 1 in]
        n224 = Select(t=T4."Enabled" ("Disabled"), s=w361, f=T4."Disabled and Grayed Out" ("Disabled")) -> (s? t:f=w360:T4)
        n225 = property on="d1_A2" class="Str"("DisabledEnum"=w360) -> ()  [unwired: 2 in, 2 out]
        n226 = property on="d1_A2s" class="RadioBtnsControl (strict)"("DisabledEnum"=w360) -> ()  [unwired: 2 in, 2 out]
        n227 = case shown="False" w361 {
          frame False {
            w364 = FALSE ("Plot.Visible")
            n228 = property on="Graphs hP" class="WFChart (strict)"("Active Plot"=u32 1) -> (error out=w368:errorcluster)  [unwired: 2 in, 1 out]
            n229 = property on="Graphs lP" class="WFChart (strict)"("Active Plot"=u32 1) -> (error out=w365:errorcluster)  [unwired: 2 in, 1 out]
            n230 = property on="Graphs hP" class="WFChart (strict)"(error in=w368, "Plot.Visible?"=w364) -> ()  [unwired: 1 in, 2 out]
            n231 = property on="Graphs lP" class="WFChart (strict)"(error in=w365, "Plot.Visible?"=w364) -> ()  [unwired: 1 in, 2 out]
          }
          frame True {
            n232 = local read "d1_A2s"() -> (w369:enum32{"Radio Selection 1", "Radio Selection 2"})
            n233 = property on="d1_A2s" class="RadioBtnsControl (strict)"("Val(Sgnl)"=w369) -> ()  [unwired: 2 in, 2 out]
          }
        }
      }
      event "1_B1": Value Change {
        n234 = event-data() -> ("NewVal"=w371:bool)  [unwired: 1 in]
        n235 = Select(t=T4."Enabled" ("Disabled"), s=w371, f=T4."Disabled and Grayed Out" ("Disabled")) -> (s? t:f=w370:T4)
        n236 = property on="d1_B1" class="Str"("DisabledEnum"=w370) -> ()  [unwired: 2 in, 2 out]
        n237 = property on="d1_B1s" class="RadioBtnsControl (strict)"("DisabledEnum"=w370) -> ()  [unwired: 2 in, 2 out]
        n238 = case shown="False" w371 {
          frame False {
            w374 = FALSE ("Plot.Visible")
            n239 = property on="Graphs hP" class="WFChart (strict)"("Active Plot"=u32 2) -> (error out=w378:errorcluster)  [unwired: 2 in, 1 out]
            n240 = property on="Graphs lP" class="WFChart (strict)"("Active Plot"=u32 2) -> (error out=w375:errorcluster)  [unwired: 2 in, 1 out]
            n241 = property on="Graphs hP" class="WFChart (strict)"(error in=w378, "Plot.Visible?"=w374) -> ()  [unwired: 1 in, 2 out]
            n242 = property on="Graphs lP" class="WFChart (strict)"(error in=w375, "Plot.Visible?"=w374) -> ()  [unwired: 1 in, 2 out]
          }
          frame True {
            n243 = local read "d1_B1s"() -> (w379:enum32{"Radio Selection 1", "Radio Selection 2"})
            n244 = property on="d1_B1s" class="RadioBtnsControl (strict)"("Val(Sgnl)"=w379) -> ()  [unwired: 2 in, 2 out]
          }
        }
      }
      event "1_B2": Value Change {
        n245 = event-data() -> ("NewVal"=w381:bool)  [unwired: 1 in]
        n246 = Select(t=T4."Enabled" ("Disabled"), s=w381, f=T4."Disabled and Grayed Out" ("Disabled")) -> (s? t:f=w380:T4)
        n247 = property on="d1_B2" class="Str"("DisabledEnum"=w380) -> ()  [unwired: 2 in, 2 out]
        n248 = property on="d1_B2s" class="RadioBtnsControl (strict)"("DisabledEnum"=w380) -> ()  [unwired: 2 in, 2 out]
        n249 = case shown="False" w381 {
          frame False {
            w384 = FALSE ("Plot.Visible")
            n250 = property on="Graphs hP" class="WFChart (strict)"("Active Plot"=u32 3) -> (error out=w388:errorcluster)  [unwired: 2 in, 1 out]
            n251 = property on="Graphs lP" class="WFChart (strict)"("Active Plot"=u32 3) -> (error out=w385:errorcluster)  [unwired: 2 in, 1 out]
            n252 = property on="Graphs hP" class="WFChart (strict)"(error in=w388, "Plot.Visible?"=w384) -> ()  [unwired: 1 in, 2 out]
            n253 = property on="Graphs lP" class="WFChart (strict)"(error in=w385, "Plot.Visible?"=w384) -> ()  [unwired: 1 in, 2 out]
          }
          frame True {
            n254 = local read "d1_B2s"() -> (w389:enum32{"Radio Selection 1", "Radio Selection 2"})
            n255 = property on="d1_B2s" class="RadioBtnsControl (strict)"("Val(Sgnl)"=w389) -> ()  [unwired: 2 in, 2 out]
          }
        }
      }
      event "2_A1": Value Change {
        n256 = event-data() -> ("NewVal"=w391:bool)  [unwired: 1 in]
        n257 = Select(t=T4."Enabled" ("Disabled"), s=w391, f=T4."Disabled and Grayed Out" ("Disabled")) -> (s? t:f=w390:T4)
        n258 = property on="d2_A1" class="Str"("DisabledEnum"=w390) -> ()  [unwired: 2 in, 2 out]
        n259 = property on="d2_A1s" class="RadioBtnsControl (strict)"("DisabledEnum"=w390) -> ()  [unwired: 2 in, 2 out]
        n260 = case shown="False" w391 {
          frame False {
            w394 = FALSE ("Plot.Visible")
            n261 = property on="Graphs hP" class="WFChart (strict)"("Active Plot"=u32 4) -> (error out=w398:errorcluster)  [unwired: 2 in, 1 out]
            n262 = property on="Graphs lP" class="WFChart (strict)"("Active Plot"=u32 4) -> (error out=w395:errorcluster)  [unwired: 2 in, 1 out]
            n263 = property on="Graphs hP" class="WFChart (strict)"(error in=w398, "Plot.Visible?"=w394) -> ()  [unwired: 1 in, 2 out]
            n264 = property on="Graphs lP" class="WFChart (strict)"(error in=w395, "Plot.Visible?"=w394) -> ()  [unwired: 1 in, 2 out]
          }
          frame True {
            n265 = local read "d2_A1s"() -> (w399:enum32{"Radio Selection 1", "Radio Selection 2"})
            n266 = property on="d2_A1s" class="RadioBtnsControl (strict)"("Val(Sgnl)"=w399) -> ()  [unwired: 2 in, 2 out]
          }
        }
      }
      event "2_A2": Value Change {
        n267 = event-data() -> ("NewVal"=w401:bool)  [unwired: 1 in]
        n268 = Select(t=T4."Enabled" ("Disabled"), s=w401, f=T4."Disabled and Grayed Out" ("Disabled")) -> (s? t:f=w400:T4)
        n269 = property on="d2_A2" class="Str"("DisabledEnum"=w400) -> ()  [unwired: 2 in, 2 out]
        n270 = property on="d2_A2s" class="RadioBtnsControl (strict)"("DisabledEnum"=w400) -> ()  [unwired: 2 in, 2 out]
        n271 = case shown="False" w401 {
          frame False {
            w404 = FALSE ("Plot.Visible")
            n272 = property on="Graphs hP" class="WFChart (strict)"("Active Plot"=u32 5) -> (error out=w408:errorcluster)  [unwired: 2 in, 1 out]
            n273 = property on="Graphs lP" class="WFChart (strict)"("Active Plot"=u32 5) -> (error out=w405:errorcluster)  [unwired: 2 in, 1 out]
            n274 = property on="Graphs hP" class="WFChart (strict)"(error in=w408, "Plot.Visible?"=w404) -> ()  [unwired: 1 in, 2 out]
            n275 = property on="Graphs lP" class="WFChart (strict)"(error in=w405, "Plot.Visible?"=w404) -> ()  [unwired: 1 in, 2 out]
          }
          frame True {
            n276 = local read "d2_A2s"() -> (w409:enum32{"Radio Selection 1", "Radio Selection 2"})
            n277 = property on="d2_A2s" class="RadioBtnsControl (strict)"("Val(Sgnl)"=w409) -> ()  [unwired: 2 in, 2 out]
          }
        }
      }
      event "2_B1": Value Change {
        n278 = event-data() -> ("NewVal"=w411:bool)  [unwired: 1 in]
        n279 = Select(t=T4."Enabled" ("Disabled"), s=w411, f=T4."Disabled and Grayed Out" ("Disabled")) -> (s? t:f=w410:T4)
        n280 = property on="d2_B1s" class="RadioBtnsControl (strict)"("DisabledEnum"=w410) -> ()  [unwired: 2 in, 2 out]
        n281 = property on="d2_B1" class="Str"("DisabledEnum"=w410) -> ()  [unwired: 2 in, 2 out]
        n282 = case shown="False" w411 {
          frame False {
            w414 = FALSE ("Plot.Visible")
            n283 = property on="Graphs hP" class="WFChart (strict)"("Active Plot"=u32 6) -> (error out=w418:errorcluster)  [unwired: 2 in, 1 out]
            n284 = property on="Graphs lP" class="WFChart (strict)"("Active Plot"=u32 6) -> (error out=w415:errorcluster)  [unwired: 2 in, 1 out]
            n285 = property on="Graphs hP" class="WFChart (strict)"(error in=w418, "Plot.Visible?"=w414) -> ()  [unwired: 1 in, 2 out]
            n286 = property on="Graphs lP" class="WFChart (strict)"(error in=w415, "Plot.Visible?"=w414) -> ()  [unwired: 1 in, 2 out]
          }
          frame True {
            n287 = local read "d2_B1s"() -> (w419:enum32{"Radio Selection 1", "Radio Selection 2"})
            n288 = property on="d2_B1s" class="RadioBtnsControl (strict)"("Val(Sgnl)"=w419) -> ()  [unwired: 2 in, 2 out]
          }
        }
      }
      event "2_B2": Value Change {
        n289 = event-data() -> ("NewVal"=w421:bool)  [unwired: 1 in]
        n290 = Select(t=T4."Enabled" ("Disabled"), s=w421, f=T4."Disabled and Grayed Out" ("Disabled")) -> (s? t:f=w420:T4)
        n291 = property on="d2_B2s" class="RadioBtnsControl (strict)"("DisabledEnum"=w420) -> ()  [unwired: 2 in, 2 out]
        n292 = property on="d2_B2" class="Str"("DisabledEnum"=w420) -> ()  [unwired: 2 in, 2 out]
        n293 = case shown="False" w421 {
          frame False {
            w424 = FALSE ("Plot.Visible")
            n294 = property on="Graphs hP" class="WFChart (strict)"("Active Plot"=u32 7) -> (error out=w428:errorcluster)  [unwired: 2 in, 1 out]
            n295 = property on="Graphs lP" class="WFChart (strict)"("Active Plot"=u32 7) -> (error out=w425:errorcluster)  [unwired: 2 in, 1 out]
            n296 = property on="Graphs hP" class="WFChart (strict)"(error in=w428, "Plot.Visible?"=w424) -> ()  [unwired: 1 in, 2 out]
            n297 = property on="Graphs lP" class="WFChart (strict)"(error in=w425, "Plot.Visible?"=w424) -> ()  [unwired: 1 in, 2 out]
          }
          frame True {
            n298 = local read "d2_B2s"() -> (w429:enum32{"Radio Selection 1", "Radio Selection 2"})
            n299 = property on="d2_B2s" class="RadioBtnsControl (strict)"("Val(Sgnl)"=w429) -> ()  [unwired: 2 in, 2 out]
          }
        }
      }
      event "port1", "D1 IP", "D2 IP", "port2": Value Change {
        w433 = T1 0 items=["no dialog", "OK message", "continue or stop message", "OK message + warnings", "continue/stop + warnings"] ("type of dialog (OK msg:1)")
        n300 = event-data() -> ()  [unwired: 1 in, 1 out]
        n301 = local read "d1_A1s"() -> (w431:enum32{"Radio Selection 1", "Radio Selection 2"})
        n302 = local read "d2_B2s"() -> (w430:enum32{"Radio Selection 1", "Radio Selection 2"})
        n303 = call "Read and Write Controls to Automatic Config File.vi"("Action"=RWC_Actions."Write", "Control References"=w432) -> ("error out"=w434:errorcluster)  [unwired: 9 in]
        n304 = property on="d1_A1s" class="RadioBtnsControl (strict)"("Val(Sgnl)"=w431) -> ()  [unwired: 2 in, 2 out]
        n305 = property on="d2_B2s" class="RadioBtnsControl (strict)"("Val(Sgnl)"=w430) -> ()  [unwired: 2 in, 2 out]
        n306 = call <vilib>:"General Error Handler.vi"("type of dialog (OK msg:1)"=w433, "error in (no error)"=w434) -> ()  [unwired: 1 in, 13 out]
      }
    }
    n307 = Wait Until Next ms Multiple(millisecond multiple=u32 100) -> ()  [unwired: 1 out]
    n308 = local read "stop"() -> (w236:bool)
  }
  n309 = property on="P max hp" class="DigNum (strict)"("DisabledEnum"=w11) -> ()  [unwired: 2 in, 2 out]
  n310 = property on="P min hp" class="DigNum (strict)"("DisabledEnum"=w11) -> ()  [unwired: 2 in, 2 out]
  n311 = property on="P max lp" class="DigNum (strict)"("DisabledEnum"=w10) -> ()  [unwired: 2 in, 2 out]
  n312 = property on="P min lp" class="DigNum (strict)"("DisabledEnum"=w10) -> ()  [unwired: 2 in, 2 out]
  n313 = call "Read and Write Controls to Automatic Config File.vi"("Action"=RWC_Actions."Read", "Control References"=w1) -> ("error out"=w7:errorcluster)  [unwired: 9 in]
  n314 = invoke on="Graphs hP" class="WFChart (strict)" method="Reinit To Default"() -> ()  [unwired: 3 in, 3 out]
  n315 = invoke on="Graphs lP" class="WFChart (strict)" method="Reinit To Default"() -> ()  [unwired: 3 in, 3 out]
  n316 = call <vilib>:"General Error Handler.vi"("type of dialog (OK msg:1)"=w6, "error in (no error)"=w7) -> ()  [unwired: 1 in, 13 out]
  n317 = property on="Graphs hP" class="WFChart (strict)"("YScale.ScaleFit"=w9) -> ()  [unwired: 2 in, 2 out]
  n318 = property on="Graphs lP" class="WFChart (strict)"("YScale.ScaleFit"=w9) -> ()  [unwired: 2 in, 2 out]
  n319 = property on="Graphs lP" class="WFChart (strict)"("History Data"=w12) -> ()  [unwired: 2 in, 2 out]
  n320 = property on="Graphs hP" class="WFChart (strict)"("History Data"=w12) -> ()  [unwired: 2 in, 2 out]
